vi "Area.vi"(8 "error in (no error)":errorcluster, 11 "Triangle in":refnum<class "Triangle.lvclass">) -> (0 "error out":errorcluster, 2 "rect":T1, 3 "Triangle out":refnum<class "Triangle.lvclass">)   [LabVIEW 2021, in "Picture2D.lvlib" / "Triangle.lvclass"]
uses:
  Triangle.lvclass
  Point/Point.lvclass
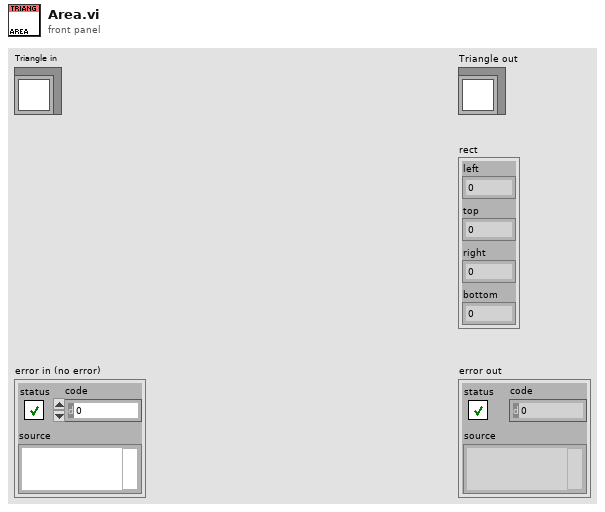
[diagram p1: front panel]
types:
  T1 = cluster{"left":i16, "top":i16, "right":i16, "bottom":i16}
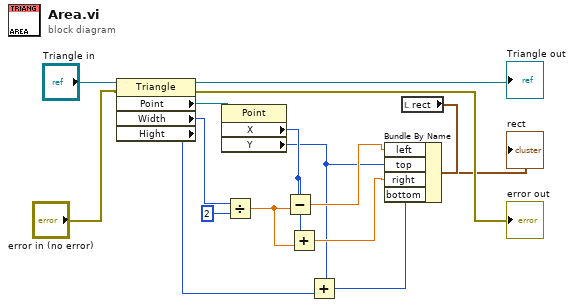
[diagram p0: block diagram]
diagram:
  n1 = property class="Triangle"(reference="Triangle in", error in="error in (no error)") -> (reference out=→"Triangle out":refnum<class "Triangle.lvclass">, error out=→"error out":errorcluster, "Point"=w14:refnum<class "Point.lvclass">, "Width"=w9:i16, "Hight"=w2:i16)
  n2 = property class="Point"(reference=w14) -> ("X"=w6:i16, "Y"=w3:i16)  [unwired: 1 in, 2 out]
  n3 = Divide(x=w9, y=i16 2) -> (x/y=w4:dbl)
  n4 = Subtract(x=w6, y=w4) -> (x-y=w7:dbl)
  n5 = Add(x=w6, y=w4) -> (x+y=w5:dbl)
  n6 = Add(x=w3, y=w2) -> (x+y=w1:i16)
  n7 = local read "rect"() -> (w11:T1)
  n8 = Bundle By Name(cluster=w11, "left"=w7, "top"=w3, "right"=w5, "bottom"=w1) -> (→"rect":T1)
